vi "Add_dummy_channels.vi"(1 "Ch & spans":T1[](array[typedef]) {"low limit (-10V)" format="%.3f"; "high limit (10V)" format="%.3f"}) -> (0 "Ch & spans":T1[](array[typedef]) {"low limit (-10V)" format="%.3f"; "high limit (10V)" format="%.3f"})   [LabVIEW 2010]
uses:
  Controls/Ch_and_Spans.ctl
panel:
  out "Unused ch No":i32[](array[numeric])
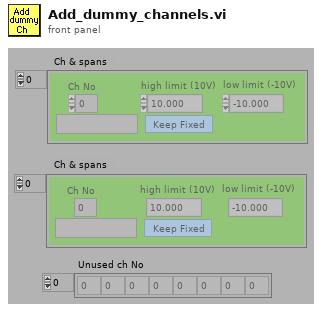
[diagram p1: front panel]
types:
  T1 = typedef "Ch_and_Spans.ctl" = cluster{"high limit (10V)":sgl, "low limit (-10V)":sgl, "Ch No":i16, "Var name":string, "Use Latest Calib":bool}
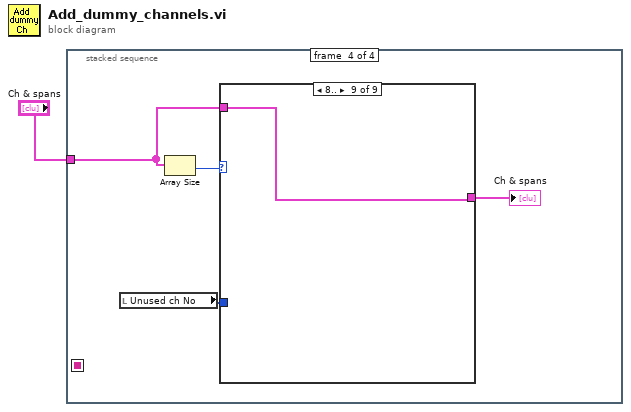
[diagram p0: block diagram]
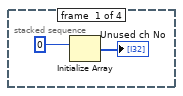
[diagram p2: hidden frame]
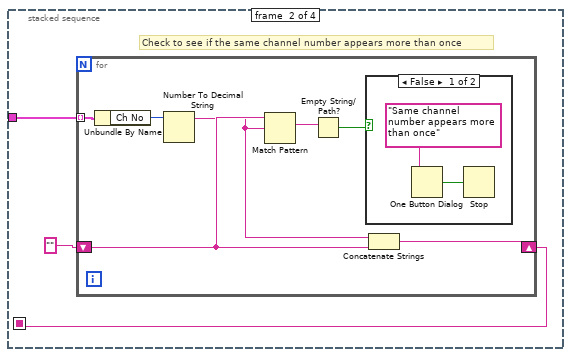
[diagram p3: hidden frame]
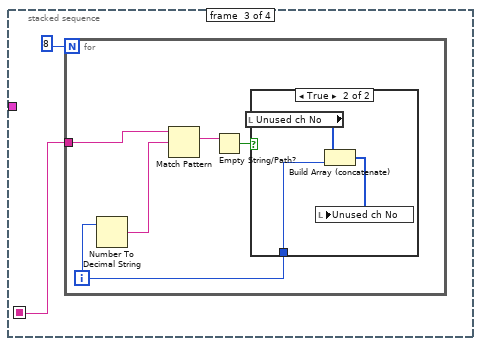
[diagram p5: hidden frame]
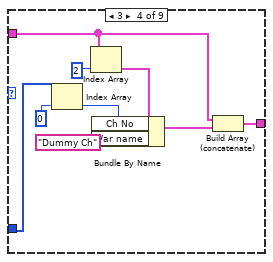
[diagram p10: hidden frame]
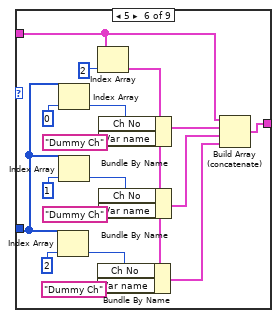
[diagram p12: hidden frame]
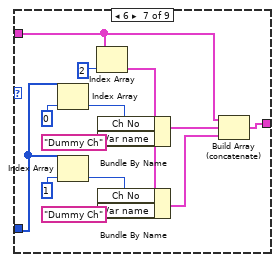
[diagram p13: hidden frame]
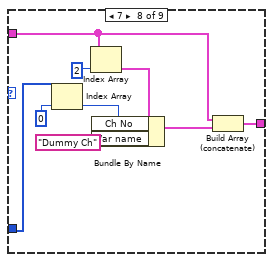
[diagram p14: hidden frame]
diagram:
  n1 = stacked-sequence {
    seq-local: [_ w4 _ _] -> [_ _ w16 _]
    tunnel: "Ch & spans" -> [_ w5 _ w28]
    frame #0 {
      n2 = Initialize Array(0) -> (→"Unused ch No":i32[])  [unwired: 1 out]
    }
    frame #1 {
      # "Check to see if the same channel number appears more than once"
      n3 = for {
        tunnel: w5 -> [w13] mode=indexing
        shift-right: [w11] -> w4
        shift-left: "" -> [w10]
        n4 = Unbundle By Name(w13) -> ("Ch No"=w12:i16)
        n5 = Number To Decimal String(number=w12) -> (decimal integer string=w9:string)  [unwired: 1 out]
        n6 = Match Pattern(string=w10, regular expression=w9) -> (match substring=w8:string)  [unwired: 4 out]
        n7 = Empty String/Path?(string/path=w8) -> (empty?=w7:bool)
        n8 = case shown="False" w7 {
          frame False {
            n9 = One Button Dialog(message="Same channel number appears more than once") -> (true=w15:bool)  [unwired: 1 out]
            n10 = Stop(stop? (T)=w15) -> ()
          }
          frame True {
          }
        }
        n11 = Concatenate Strings(w9, w10) -> (w11:string)
      }
    }
    frame #2 {
      n12 = for {
        N: 8 -> [_]
        tunnel: w16 -> [w22]
        i -> [w21]
        n13 = Number To Decimal String(number=w21) -> (decimal integer string=w20:string)  [unwired: 1 out]
        n14 = Match Pattern(string=w22, regular expression=w20) -> (match substring=w19:string)  [unwired: 4 out]
        n15 = Empty String/Path?(string/path=w19) -> (empty?=w18:bool)
        n16 = case shown="True" w18 {
          tunnel: w21 -> [_ w24]
          frame False {
          }
          frame True {
            n17 = local read "Unused ch No"() -> (w25:i32[])
            n18 = Build Array (concatenate)(w25, w24) -> (w23:i32[])
            n19 = local write "Unused ch No"(w23) -> ()
          }
        }
      }
    }
    frame #3 {
      n20 = local read "Unused ch No"() -> (w26:i32[])
      n21 = Array Size(array=w28) -> (size(s)=w29:i32)
      n22 = case shown="8.." w29 {
        tunnel: w28 -> [w30 w31 w32 w39 w42 w57 w70 w79 w82]
        tunnel: [w30 w31 w32 w41 w42 w59 w72 w81 w82] -> w27
        tunnel: w26 -> [_ _ _ w33 _ w47 w63 w73 _]
        frame ..0 {
        }
        frame 1 {
        }
        frame 2 {
        }
        frame 3 {
          n23 = Index Array(array=w33, index=0) -> (element=w36:i32)
          n24 = Index Array(array=w39, index=2) -> (element=w34:T1)
          n25 = Bundle By Name(cluster=w34, "Ch No"=w36, "Var name"="Dummy Ch") -> (w35:T1)
          n26 = Build Array (concatenate)(w39, w35) -> (w41:T1[])
        }
        frame 4 {
        }
        frame 5 {
          n27 = Index Array(array=w47, index=2) -> (element=w54:i32)
          n28 = Index Array(array=w47, index=0) -> (element=w48:i32)
          n29 = Index Array(array=w47, index=1) -> (element=w53:i32)
          n30 = Index Array(array=w57, index=2) -> (element=w46:T1)
          n31 = Bundle By Name(cluster=w46, "Ch No"=w54, "Var name"="Dummy Ch") -> (w43:T1)
          n32 = Bundle By Name(cluster=w46, "Ch No"=w48, "Var name"="Dummy Ch") -> (w45:T1)
          n33 = Bundle By Name(cluster=w46, "Ch No"=w53, "Var name"="Dummy Ch") -> (w44:T1)
          n34 = Build Array (concatenate)(w57, w45, w44, w43) -> (w59:T1[])
        }
        frame 6 {
          n35 = Index Array(array=w63, index=0) -> (element=w64:i32)
          n36 = Index Array(array=w63, index=1) -> (element=w69:i32)
          n37 = Index Array(array=w70, index=2) -> (element=w62:T1)
          n38 = Bundle By Name(cluster=w62, "Ch No"=w64, "Var name"="Dummy Ch") -> (w61:T1)
          n39 = Bundle By Name(cluster=w62, "Ch No"=w69, "Var name"="Dummy Ch") -> (w60:T1)
          n40 = Build Array (concatenate)(w70, w61, w60) -> (w72:T1[])
        }
        frame 7 {
          n41 = Index Array(array=w73, index=0) -> (element=w76:i32)
          n42 = Index Array(array=w79, index=2) -> (element=w74:T1)
          n43 = Bundle By Name(cluster=w74, "Ch No"=w76, "Var name"="Dummy Ch") -> (w75:T1)
          n44 = Build Array (concatenate)(w79, w75) -> (w81:T1[])
        }
        frame 8.. {
        }
      }
      "Ch & spans" <- w27
    }
  }
